vi "Get_TemperatureStatus.vi"(8 "error in (no error)":errorcluster, 11 "Abstract_CCD in":refnum<class "Abstract_CCD.lvclass">) -> (0 "error out":errorcluster, 2 "Enum":T1(ring), 3 "Abstract_CCD out":refnum<class "Abstract_CCD.lvclass">)   [LabVIEW 2020, in "Abstract_CCD.lvclass"]
uses:
  <instrlib>/Classes/CCD/Abstract_CCD/Abstract_CCD.lvclass
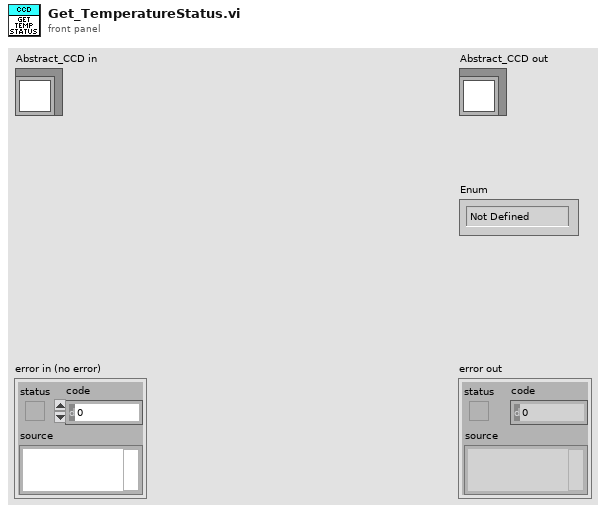
[diagram p1: front panel]
types:
  T1 = enum16{"Not Defined", "Unlocked", "Locked", "Not Reached"}
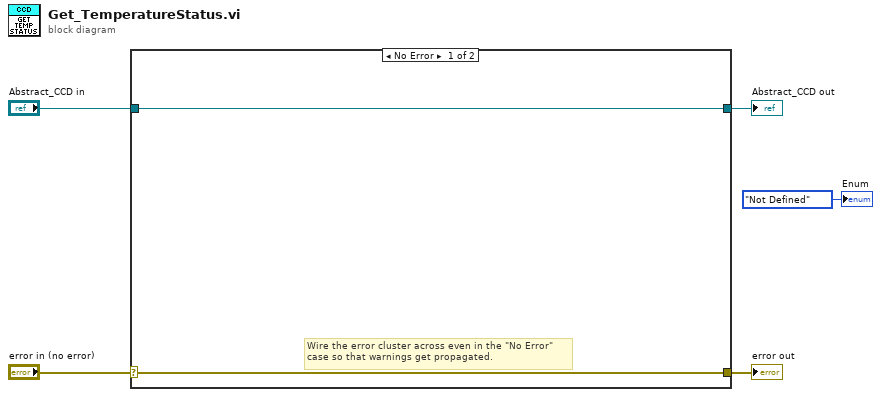
[diagram p0: block diagram]
diagram:
  n1 = case shown="No Error" "error in (no error)" {
    selector: "error in (no error)" -> [w6 w9]
    tunnel: [w6 w9] -> w4
    tunnel: [w7 w8] -> w2
    tunnel: "Abstract_CCD in" -> [w7 w8]
    frame No Error {
      # "Wire the error cluster across even in the \"No Error\"\ncase so that warnings get propagated."
    }
    frame Error {
    }
  }
  "error out" <- w4
  "Abstract_CCD out" <- w2
  "Enum" <- enum16{"Not Defined", "Unlocked", "Locked"}."Not Defined" ("Enum")
